vi "Attributes.vi"(7 "Action":enum8{"get", "set"}(ring), 8 "error in (no error)":errorcluster, 10 "Self in":T1, 11 "Instance in":variant) -> (0 "error out":errorcluster, 2 "Self out":T1, 3 "Instance out":variant)   [LabVIEW 2018, in "Core.lvlib" / "Module.lvlib"]
uses:
  Module.lvlib
  Controls/Instance.ctl
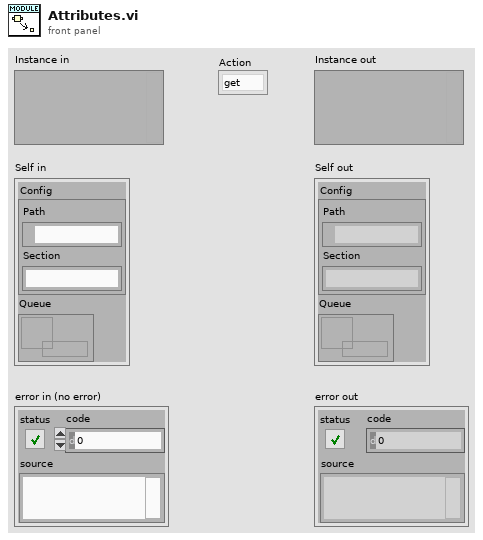
[diagram p1: front panel]
types:
  T1 = typedef "Core.lvlib/Module.lvlib/Instance.ctl" = cluster{"Config":cluster{"Path":path, "Section":string}, "Queue":refnum<queue>}
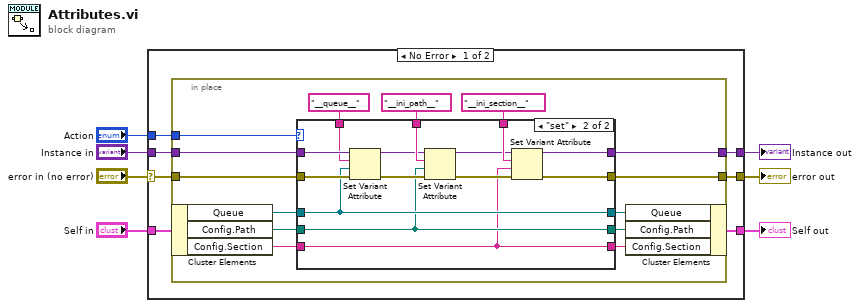
[diagram p0: block diagram]
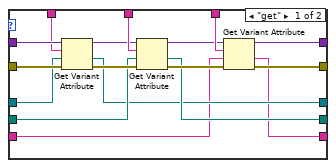
[diagram p2: hidden frame]
diagram:
  n1 = case shown="No Error" "error in (no error)" {
    selector: "error in (no error)" -> [w14 w62]
    tunnel: "Instance in" -> [w13 w61]
    tunnel: [w12 w62] -> w5
    tunnel: [w11 w61] -> w4
    tunnel: [w10 w60] -> w3
    tunnel: "Self in" -> [w9 w60]
    tunnel: "Action" -> [w8 _]
    frame No Error {
      n2 = in-place {
        in-place-border: w14 -> [w28]
        in-place-border: w13 -> [w27]
        in-place-border: [w23] -> w12
        in-place-border: [w22] -> w11
        in-place-border: w8 -> [w15]
        n3 = in-place-cluster #1(w9) -> ("Queue"=w21:refnum<queue>, "Config.Path"=w20:path, "Config.Section"=w17:string)
        n4 = case shown="\"set\"" w15 {
          tunnel: w28 -> [w45 w59]
          tunnel: w27 -> [w44 w58]
          tunnel: "__queue__" ("name") -> [w43 w57]
          tunnel: "__ini_path__" ("name") -> [w42 w56]
          tunnel: "__ini_section__" ("name") -> [w39 w53]
          tunnel: [w36 w50] -> w23
          tunnel: [w35 w49] -> w22
          tunnel: w21 -> [w34 w48]
          tunnel: w20 -> [w33 w47]
          tunnel: [w32 w47] -> w19
          tunnel: [w31 w48] -> w18
          tunnel: w17 -> [w30 w46]
          tunnel: [w29 w46] -> w16
          frame "get" {
            n5 = Get Variant Attribute(Variant=w44, name=w43, default value (empty Variant)=w34, error in=w45) -> (duplicate Variant=w41:variant, value=w31:refnum<queue>, error out=w40:errorcluster)  [unwired: 1 out]
            n6 = Get Variant Attribute(Variant=w41, name=w42, default value (empty Variant)=w33, error in=w40) -> (duplicate Variant=w38:variant, value=w32:path, error out=w37:errorcluster)  [unwired: 1 out]
            n7 = Get Variant Attribute(Variant=w38, name=w39, default value (empty Variant)=w30, error in=w37) -> (duplicate Variant=w35:variant, value=w29:string, error out=w36:errorcluster)  [unwired: 1 out]
          }
          frame "set" {
            n8 = Set Variant Attribute(Variant=w58, name=w57, value=w48, error in=w59) -> (Variant out=w55:variant, error out=w54:errorcluster)  [unwired: 1 out]
            n9 = Set Variant Attribute(Variant=w55, name=w56, value=w47, error in=w54) -> (Variant out=w52:variant, error out=w51:errorcluster)  [unwired: 1 out]
            n10 = Set Variant Attribute(Variant=w52, name=w53, value=w46, error in=w51) -> (Variant out=w49:variant, error out=w50:errorcluster)  [unwired: 1 out]
          }
        }
        n11 = in-place-cluster #1("Queue"=w18, "Config.Path"=w19, "Config.Section"=w16) -> (w10:T1)
      }
    }
    frame Error {
    }
  }
  "Instance out" <- w4
  "error out" <- w5
  "Self out" <- w3
